vi "AscIIToChar(cast).vi"(1 "ASCII":u8 format="DEC:%2d\nHEX:%2x") -> (0 "Char":string)   [LabVIEW 2012]
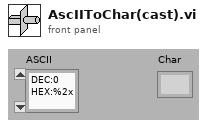
[diagram p1: front panel]
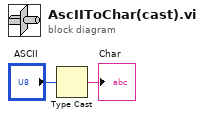
[diagram p0: block diagram]
diagram:
  n1 = Type Cast(x="ASCII") -> (*(type *) &x=→"Char":string)  [unwired: 1 in]
